vi "IOP Control_backup.vi"() -> ()   [LabVIEW 2016]
uses:
  <vilib>/Platform/TimedLoop/XDataNode/timing_clust.ctl
  <vilib>/Platform/TimedLoop/XDataNode/nitl_modes.ctl
  <vilib>/Platform/TimedLoop/XDataNode/wakeup.ctl
  <vilib>/FPGAPlugInAG/PXI-7833R/niLvFpga_Open_PXI-7833R.vi
  <vilib>/Utility/error.llb/Error Cluster From Error Code.vi
  <vilib>/rvi/errors/niLvFpgaAdjustHostInterfaceError.vi
  <vilib>/Utility/file.llb/Write Delimited Spreadsheet (string).vi
  <vilib>/Utility/file.llb/Write Delimited Spreadsheet (DBL).vi
  <vilib>/FPGAPlugInAG/PXI-7833R/niLvFpga_Reset_PXI-7833R.vi
  <vilib>/FPGAPlugInAG/PXI-7833R/niLvFpga_Close_PXI-7833R.vi
  <vilib>/rvi/interface/nirviOpenFPGA/nirviOpenFPGA.xnode
  FPGA Bitfiles/IRISSTrack_FPGATarget_IRISSFPGAIOv4_6RY0Tmt7PDg.lvbitx
  IRISS_FPGA_IO_v4.vi
  <vilib>/rvi/interface/nirviReadWriteControl/nirviReadWriteControl.xnode
  <vilib>/platform/TimedLoop/XDataNode/XDataNode.xnode
  <vilib>/rvi/interface/nirviMethod/nirviMethod.xnode
  <vilib>/rvi/interface/nirviCloseFPGA/nirviCloseFPGA.xnode
  NiFpgaLv.dll
  Library/KevinLibraryAll/labview2011/kevLib2011.lvlib
  <vilib>/Platform/TimedLoop/XDataNode/XDNodeRunTimeDep.lvlib
panel:
  out "Sensor Reading":dbl[](array[numeric]) caption="IOP Output [mmHg]"
  out "Finished Late Counts":u16
  out "Vac Cmd Indicator":dbl
  in  "Stop Vacuum?":bool
  in  "Irrigation?":bool
  in  "PID ON/OFF":bool
  in  "Vac Limit":dbl=600.0 min=0.0 max=100.0 step=1.0 format="%#_13g"
  in  "PID Gains":cluster{"Kp":dbl, "Kd":dbl, "Ki":dbl, "Ts":dbl}={"Kp"=1.0, "Kd"=0.0, "Ki"=5.0, "Ts"=0.01}
  out "Error(s) Out on Program End":errorcluster
  out "Elaspsed Time":dbl
  in  "File Path":path=path "C:/KevData1.txt"
  in  "Take Data":bool
  out "File Exists":bool
  in  "Seconds of Data":dbl=30.0
  in  "Prog Stop":bool
  out "I/A and IOP Pressure":T1(graph)
  out "Sensor Indicator":dbl[](array[numeric]) caption="Reading"
  out "Vac Cmd Chart":dbl(graph)
  out "Period [ms]":i64=10
  in  "Vac Cmd":dbl format="%#_13g"
  in  "Target IOP":dbl=30.0 min=0.0 max=100.0 step=1.0 format="%#_13g"
  # "Irrigation"
  # "Vacuum"
  # "Ant. Chamber"
  # "Vitreous"
  # "Data Saving Section"
  # "Feedback Control Section"
  # "1. PID memory release or ramp out\n2. control action direction"
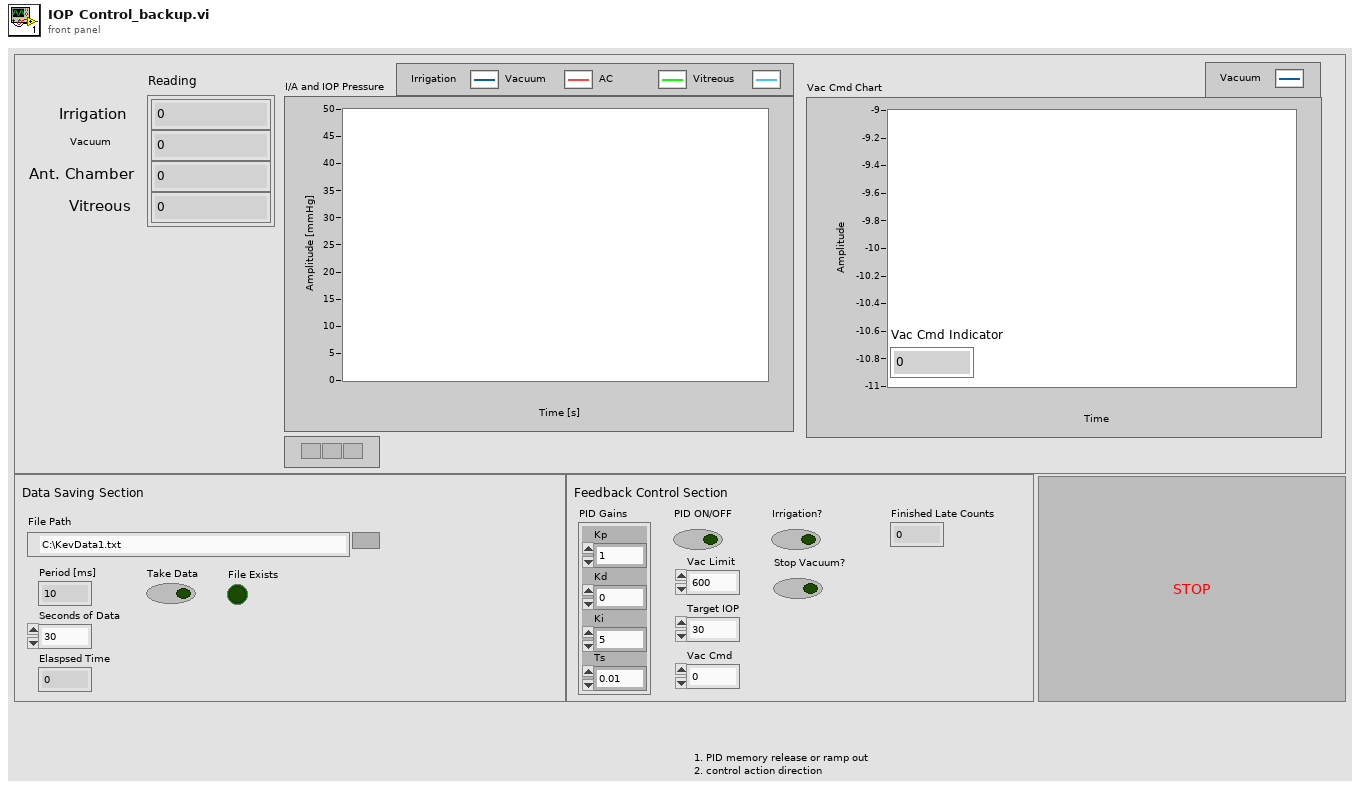
[diagram p1: front panel]
types:
  T1 = cluster{"[0]":dbl, "[1]":dbl, "[2]":dbl, "[3]":dbl, "[4]":dbl, "[5]":dbl, "[6]":dbl, "[7]":dbl, "[8]":dbl}
  T2 = typedef "XDNodeRunTimeDep.lvlib/timing_clust.ctl" = cluster{"Expected End [f-1]":u64, "Actual End [f-1]":u64, "Finished Late? [f-1]":bool, "Expected End [i-1]":u64, "Actual End [i-1]":u64, "Finished Late? [i-1]":bool, "Expected Start [i]":u64, "Actual Start [i]":u64, "Expected Start [f]":u64, "Actual Start [f]":u64, "Source Name":string, "Structure Name":string, "Period":i64, "Deadline":i64, "Offset":i64, "Start":i64, "Priority":i32, "Timeout":i32, "Mode":T3, "Wakeup Reason":T4, "Error":errorcluster, "Source Type":string, "Secondary Source Type":string, "Global End Time":u64, "Global Start Time":u64, "Frame Duration":u64, "Iteration Duration":u64, "Assigned CPU":i32, "I/O Scan Engine Mode":u32}
  T3 = typedef "XDNodeRunTimeDep.lvlib/nitl_modes.ctl" = enum32{"No Change", "Process missed periods, maintain original phase", "Discard missed periods, maintain original phase", "Process missed periods, ignore original phase", "Discard missed periods, ignore original phase"}
  T4 = typedef "XDNodeRunTimeDep.lvlib/wakeup.ctl" = enum32{"Normal", "Aborted", "Asynchronous wakeup", "Timing source error", "Timed loop error", "Timeout"}
  T5 = cluster{"Sensor Reading[0]":dbl, "Sensor Reading[1]":dbl, "Sensor Reading[2]":dbl, "Sensor Reading[3]":dbl, "Sensor Reading[4]":dbl, "Sensor Reading[5]":dbl, "Sensor Reading[6]":dbl, "Sensor Reading[7]":dbl, "Sensor Reading[8]":dbl}
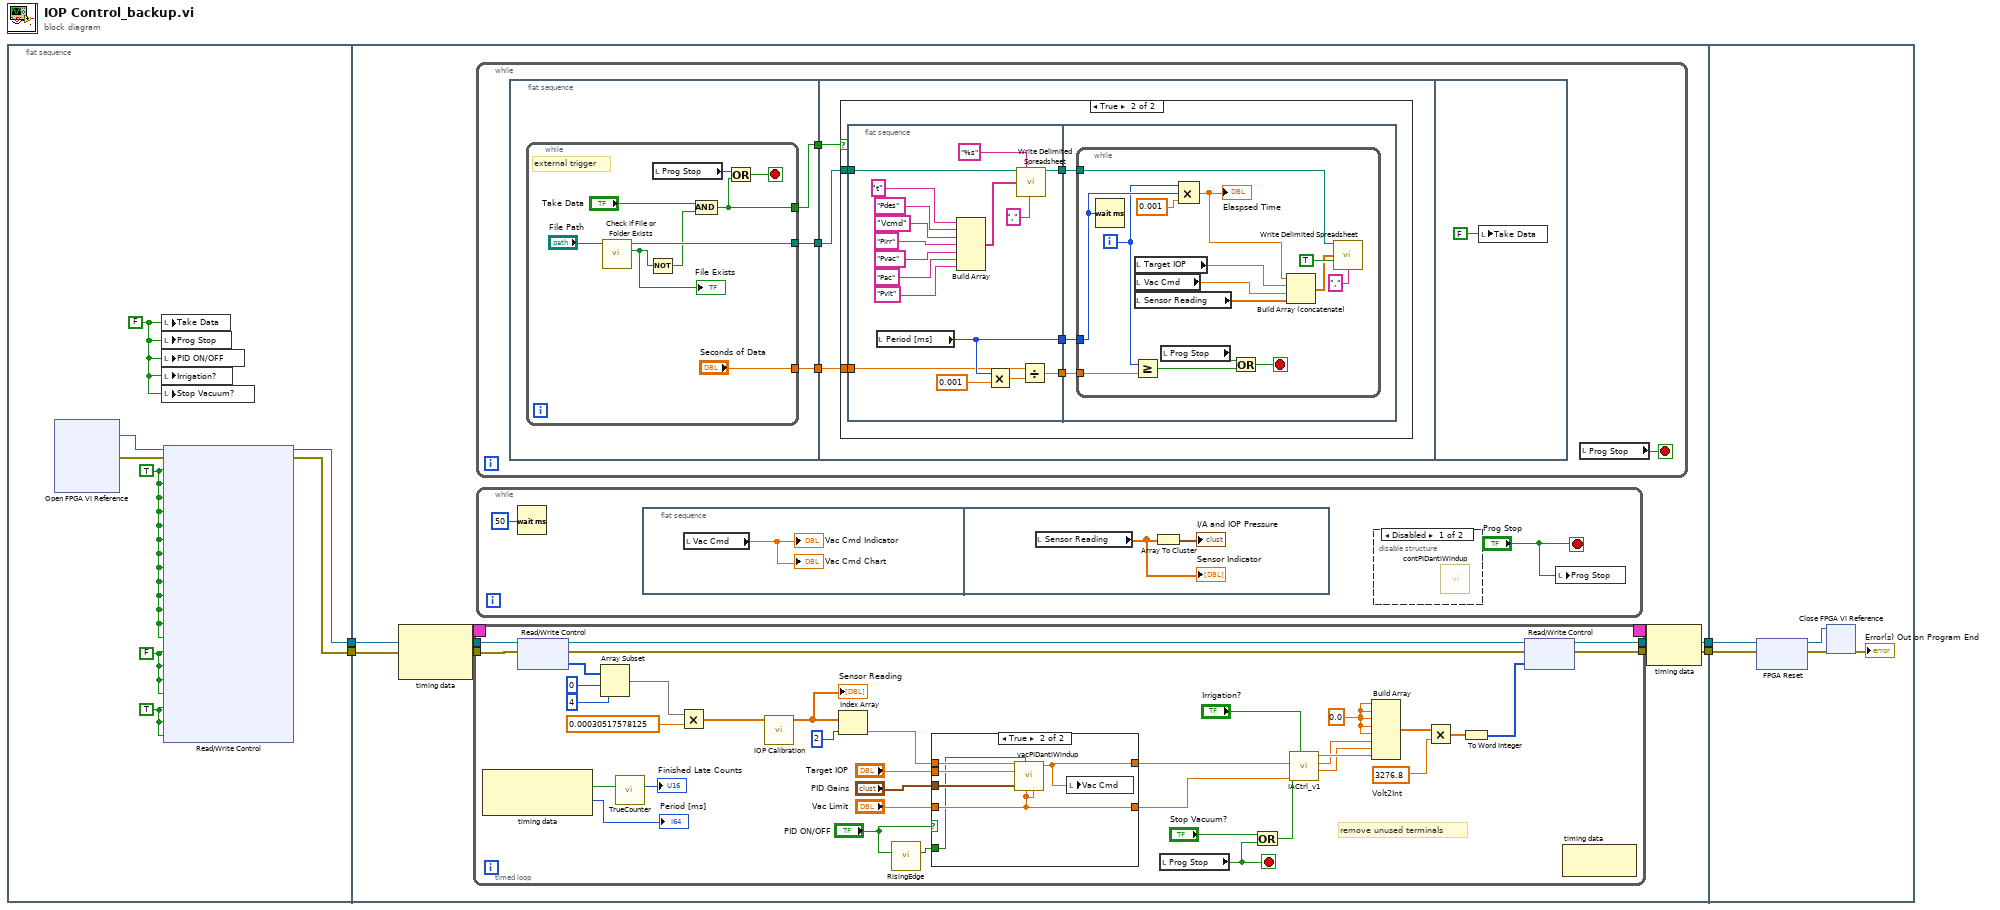
[diagram p0: block diagram]
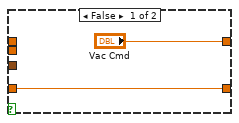
[diagram p2: hidden frame]
diagram:
  n1 = flat-sequence {
    tunnel: [w7] -> w4
    tunnel: [w6] -> w3
    tunnel: w4 -> [w18]
    tunnel: w3 -> [w17]
    tunnel: [w16] -> w2
    tunnel: [w15] -> w1
    tunnel: w2 -> [w136]
    tunnel: w1 -> [w135]
    frame #0 {
      w11 = TRUE ("Conn0/DIO12 Button 1")
      w10 = FALSE ("Reset")
      w12 = TRUE ("Reset")
      w5 = FALSE ("stop")
      n2 = xnode "Open FPGA VI Reference"() -> ("FPGA VI Reference Out"=w9:refnum<k20>, "error out"=w8:errorcluster)  [unwired: 2 in]
      n3 = local write "Take Data"(w5) -> ()
      n4 = local write "Prog Stop"(w5) -> ()
      n5 = local write "PID ON/OFF"(w5) -> ()
      n6 = local write "Irrigation?"(w5) -> ()
      n7 = local write "Stop Vacuum?"(w5) -> ()
      n8 = xnode "Read/Write Control"("FPGA VI Reference In"=w9, "error in"=w8, "Reset 1"=w12, "Reset 3"=w12, "Reset 9"=w12, "Reset 10"=w12, "Reset 11"=w12, "Reset 12"=w12, "Reset 13"=w12, "Reset 14"=w12, "Reset 15"=w12, "Reset 16"=w12, "Reset 17"=w12, "Reset C1-1"=w12, "Reset C1-4"=w12, "INHB X"=w10, "INHB Y"=w10, "INHB Z"=w10, "INHB OCT Mot"=w10, "Conn0/DIO12 Button 1"=w11, "Conn0/DIO13 Button 2"=w11, "Conn0/DIO15 Button 4"=w11) -> ("FPGA VI Reference Out"=w7:refnum<k20>, "error out"=w6:errorcluster)
    }
    frame #1 {
      n9 = node-c288() -> (w14:T2)  [unwired: 2 in]
      n10 = timed-loop {
        tunnel: w18 -> [w50]
        tunnel: w17 -> [w49]
        tunnel: [w48] -> w16
        tunnel: [w47] -> w15
        timing: w14 -> [_]
        timing-out: [_] -> w13
        stop <- w37 stop-if-true
        w34 = 0.0 ("element")
        w36 = 3276.8  # Volt2Int
        # "remove unused terminals"
        n11 = node-c288() -> (w27:bool, →"Period [ms]":i64)  [unwired: 1 in]
        n12 = xnode "Read/Write Control"("FPGA VI Reference In"=w50, "error in"=w49) -> ("FPGA VI Reference Out"=w46:refnum<k20>, "error out"=w45:errorcluster, "AI"=w55:i16[])
        n13 = Array Subset(array=w55, index=0, length=4) -> (w54:i16[])
        n14 = call "TrueCounter.vi"("True?"=w27) -> ("True Count"=→"Finished Late Counts":u16)  [unwired: 9 in]
        n15 = Multiply(x=w54, y=0.00030517578125) -> (x*y=w19:dbl[])
        n16 = call "IOP Calibration.vi"("IOP Input [V]"=w19) -> ("IOP Output [mmHg]"=w28:dbl[])  [unwired: 10 in]
        "Sensor Reading" <- w28
        n17 = Index Array(array=w28, index=2) -> (element=w23:dbl)
        n18 = call "RisingEdge.vi"("Signal In"="PID ON/OFF") -> ("Rising Edge"=w20:bool)  [unwired: 10 in]
        n19 = case shown="True" "PID ON/OFF" {
          tunnel: w23 -> [_ w63]
          tunnel: "PID Gains" -> [_ w65]
          tunnel: "Target IOP" -> [_ w64]
          tunnel: ["Vac Cmd" w67] -> w24
          tunnel: "Vac Limit" -> [w61 w66]
          tunnel: [w61 w66] -> w41
          tunnel: w20 -> [_ w62]
          frame False {
          }
          frame True {
            n20 = call "vacPIDantiWindup.vi"("Saturation U"=w66, "Saturation M"=w66, "Reset"=w62, "PID Gains"=w65, "Feedback"=w64, "Reference"=w63) -> ("Control"=w67:dbl)  [unwired: 5 in]
            n21 = local write "Vac Cmd"(w67) -> ()
          }
        }
        n22 = local read "Prog Stop"() -> (w37:bool)
        n23 = Or(x="Stop Vacuum?", y=w37) -> (x .or. y?=w39:bool)
        n24 = call "IACtrl_v1.vi"("Irrigate?"="Irrigation?", "Max Limit [mmHg]"=w41, "E-Stop Vacuum"=w39, "Vacuum Force [mmHg]"=w24) -> ("Accurus ChB Vout"=w30:dbl, "Accurus ChA Vout"=w31:dbl, "Accurus Engaged Vout"=w32:dbl)  [unwired: 2 in, 3 out]
        n25 = Build Array(w34, w34, w34, w34, w34, w31, w30, w32) -> (w33:dbl[])
        n26 = Multiply(x=w33, y=w36) -> (x*y=w35:dbl[])
        n27 = To Word Integer(number=w35) -> (16bit integer=w29:i16[])
        n28 = xnode "Read/Write Control"("FPGA VI Reference In"=w46, "error in"=w45, "AO"=w29) -> ("FPGA VI Reference Out"=w48:refnum<k20>, "error out"=w47:errorcluster)
        n29 = node-c288() -> ()  [unwired: 1 in, 1 out]
      }
      n30 = while {
        stop <- w75 stop-if-true
        n31 = flat-sequence {
          tunnel: [w79] -> w78
          tunnel: [w81] -> w77
          tunnel: [w80] -> w76
          tunnel: w78 -> [w93]
          tunnel: w77 -> [w92]
          tunnel: w76 -> [w91]
          frame #0 {
            n32 = while {
              tunnel: [w86] -> w81
              tunnel: ["Seconds of Data"] -> w80
              tunnel: [w82] -> w79
              stop <- w90 stop-if-true
              # "external trigger"
              n33 = call <vilib>:"Check if File or Folder Exists.vi"("path"="File Path") -> ("file or folder exists?"=w85:bool, "dup path"=w86:path)  [unwired: 8 in, 1 out]
              "File Exists" <- w85
              n34 = Not(x=w85) -> (.not. x?=w84:bool)
              n35 = local read "Prog Stop"() -> (w88:bool)
              n36 = And(x="Take Data", y=w84) -> (x .and. y?=w82:bool)
              n37 = Or(x=w88, y=w82) -> (x .or. y?=w90:bool)
            }
          }
          frame #1 {
            n38 = case shown="True" w93 {
              tunnel: w92 -> [_ w98]
              tunnel: w91 -> [_ w95]
              frame False {
              }
              frame True {
                n39 = flat-sequence {
                  tunnel: w98 -> [w104]
                  tunnel: [w102] -> w97
                  tunnel: [w113] -> w96
                  tunnel: w95 -> [w112]
                  tunnel: [w110] -> w94
                  tunnel: w97 -> [w118]
                  tunnel: w96 -> [w117]
                  tunnel: w94 -> [w116]
                  frame #0 {
                    n40 = local read "Period [ms]"() -> (w113:i64)
                    n41 = Build Array("t" ("delimiter (\\t)"), "Pdes" ("delimiter (\\t)"), "Vcmd" ("delimiter (\\t)"), "Pirr" ("delimiter (\\t)"), "Pvac" ("delimiter (\\t)"), "Pac" ("delimiter (\\t)"), "Pvit" ("delimiter (\\t)")) -> (w101:string[])
                    n42 = Multiply(x=w113, y=0.001) -> (x*y=w111:dbl)
                    n43 = call-poly <vilib>:"Write Delimited Spreadsheet.vi"("file path (dialog if empty)"=w104, "format (%s)"="%s", "1D data"=w101, "delimiter (\\t)"="," ("delimiter (\\t)")) -> ("new file path (Not A Path if cancelled)"=w102:path)  [unwired: 10 in, 1 out]
                    n44 = Divide(x=w112, y=w111) -> (x/y=w110:dbl)
                  }
                  frame #1 {
                    n45 = while {
                      tunnel: w118 -> [w125]
                      tunnel: w117 -> [w130]
                      tunnel: w116 -> [w128]
                      i -> [w129]
                      stop <- w132 stop-if-true
                      n46 = Wait (ms)(milliseconds to wait=w130) -> ()  [unwired: 1 out]
                      n47 = Greater Or Equal?(x=w129, y=w128) -> (x >= y?=w127:bool)
                      n48 = local read "Target IOP"() -> (w120:dbl)
                      n49 = local read "Vac Cmd"() -> (w121:dbl)
                      n50 = local read "Sensor Reading"() -> (w126:dbl[])
                      n51 = local read "Prog Stop"() -> (w133:bool)
                      n52 = Compound Arithmetic op=MULTIPLY(w129, w130, 0.001 ("y")) -> (w119:dbl)
                      "Elaspsed Time" <- w119
                      n53 = Or(x=w133, y=w127) -> (x .or. y?=w132:bool)
                      n54 = Build Array (concatenate)(w119, w120, w121, w126) -> (w123:dbl[])
                      n55 = call-poly <vilib>:"Write Delimited Spreadsheet.vi"("file path (dialog if empty)"=w125, "1D data"=w123, "append to file? (new file:F)"=TRUE, "delimiter (\\t)"="," ("delimiter (\\t)")) -> ()  [unwired: 10 in, 2 out]
                    }
                  }
                }
              }
            }
          }
          frame #2 {
            n56 = local write "Take Data"(FALSE) -> ()
          }
        }
        n57 = local read "Prog Stop"() -> (w75:bool)
      }
      n58 = while {
        stop <- "Prog Stop" stop-if-true
        n59 = Wait (ms)(milliseconds to wait=u32 50) -> ()  [unwired: 1 out]
        n60 = flat-sequence {
          frame #0 {
            n61 = local read "Vac Cmd"() -> (→"Vac Cmd Chart" →"Vac Cmd Indicator":dbl)
          }
          frame #1 {
            n62 = local read "Sensor Reading"() -> (w74:dbl[])
            "Sensor Indicator" <- w74
            n63 = Array To Cluster(array=w74) -> (cluster=→"I/A and IOP Pressure":T5)
          }
        }
        n64 = disable-structure shown="Disabled" {
          frame Disabled {
            n65 = call "contPIDantiWindup.vi"() -> ()  [unwired: 11 in, 1 out]
          }
          frame Enabled {
          }
        }
        n66 = local write "Prog Stop"("Prog Stop") -> ()
      }
      n67 = node-c288(w13) -> ()  [unwired: 1 out]
    }
    frame #2 {
      n68 = xnode "FPGA Reset"("FPGA VI Reference In"=w136, "error in"=w135) -> ("FPGA VI Reference Out"=w139:refnum<k20>, "error out"=w138:errorcluster)
      n69 = xnode "Close FPGA VI Reference"("FPGA VI Reference In"=w139, "error in"=w138) -> ("error out"=→"Error(s) Out on Program End":errorcluster)
    }
  }
